vi "Timer FGV.vi"(8 "error in":errorcluster, 10 "Timing (s)":u32, 11 "Timer Action":T1) -> (0 "error out":errorcluster, 2 "Done?":bool, 3 "Elapsed Time":dbl)   [LabVIEW 8.6]
doc: "This functional global is used to keep track of the elapsed time in a given sequence step."
uses:
  Controls/Timer Actions.ctl
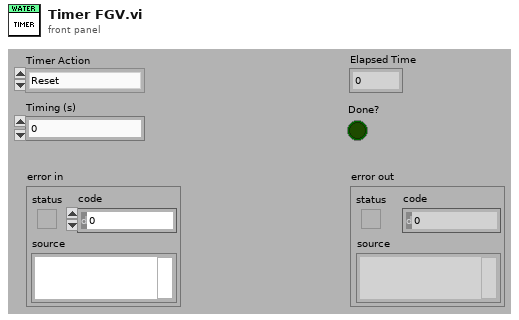
[diagram p1: front panel]
types:
  T1 = typedef "Timer Actions.ctl" = enum16{"Reset", "Check Time"}
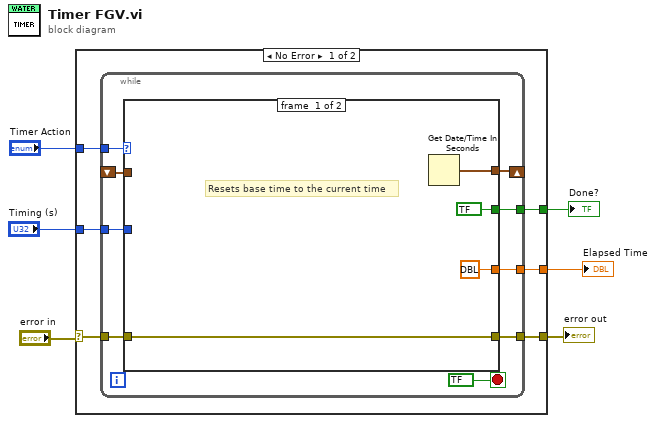
[diagram p0: block diagram]
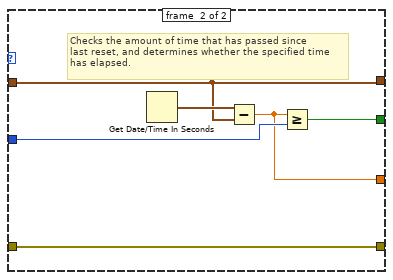
[diagram p2: hidden frame]
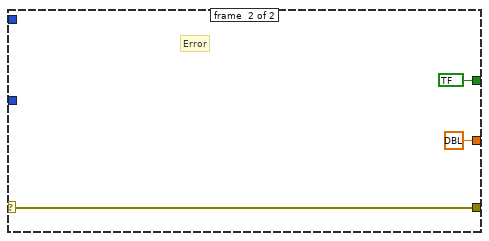
[diagram p3: hidden frame]
diagram:
  n1 = case shown="No Error" "error in" {
    selector: "error in" -> [w12 w34]
    tunnel: [w7 w34] -> w5
    tunnel: "Timer Action" -> [w11 _]
    tunnel: "Timing (s)" -> [w10 _]
    tunnel: [w9 dbl ?] -> w2
    tunnel: [w8 bool ?] -> w1
    frame #0 {
      n2 = while {
        tunnel: w12 -> [w13]
        tunnel: w11 -> [w20]
        tunnel: w10 -> [w19]
        shift-right: [w18] -> _
        shift-left: _ -> [w15]
        tunnel: [w17] -> w9
        tunnel: [w16] -> w8
        tunnel: [w14] -> w7
        stop <- bool ? stop-if-true
        n3 = case shown="\"Check Time\"" w20 {
          tunnel: w19 -> [_ w28]
          tunnel: [w25 w30] -> w18
          tunnel: [dbl ? w26] -> w17
          tunnel: [bool ? w27] -> w16
          tunnel: w15 -> [_ w30]
          tunnel: [w22 w29] -> w14
          tunnel: w13 -> [w22 w29]
          frame #0 {
            # "Resets base time to the current time"
            n4 = Get Date/Time In Seconds() -> (seconds since 1Jan1904=w25:timestamp)
          }
          frame #1 {
            # "Checks the amount of time that has passed since\nlast reset, and determines whether the specified time\nhas elapsed."
            n5 = Get Date/Time In Seconds() -> (seconds since 1Jan1904=w31:timestamp)
            n6 = Subtract(x=w31, y=w30) -> (x-y=w26:dbl)
            n7 = Greater Or Equal?(x=w26, y=w28) -> (x >= y?=w27:bool)
          }
        }
      }
    }
    frame #1 {
      # "Error"
    }
  }
  "error out" <- w5
  "Elapsed Time" <- w2
  "Done?" <- w1
